vi "Read Instrument Configuration.vi"(8 "error in":errorcluster, 10 "Module Name":string, 11 "Instrument Config File Path":path) -> (0 "error out":errorcluster, 2 "Instrument Config":T1)   [LabVIEW 2023, in "Instrument Config.lvlib"]
uses:
  Instrument Config.lvlib
  <vilib>/Utility/config.llb/Read Key (String).vi
  <vilib>/Utility/config.llb/NI_LVConfig.lvlib
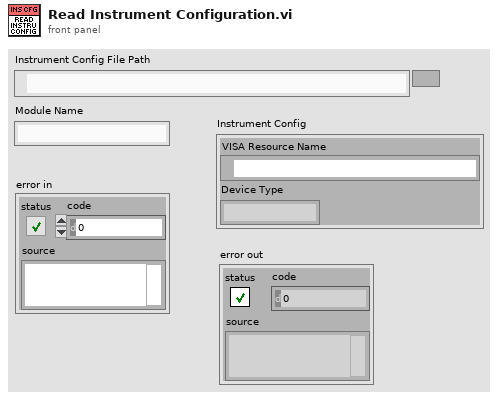
[diagram p1: front panel]
types:
  T1 = cluster{"VISA Resource Name":refnum<visa-resource-name>, "Device Type":string}
  T2 = typedef "NI_LVConfig.lvlib/Config Data RefNum.ctl" = refnum<k1>
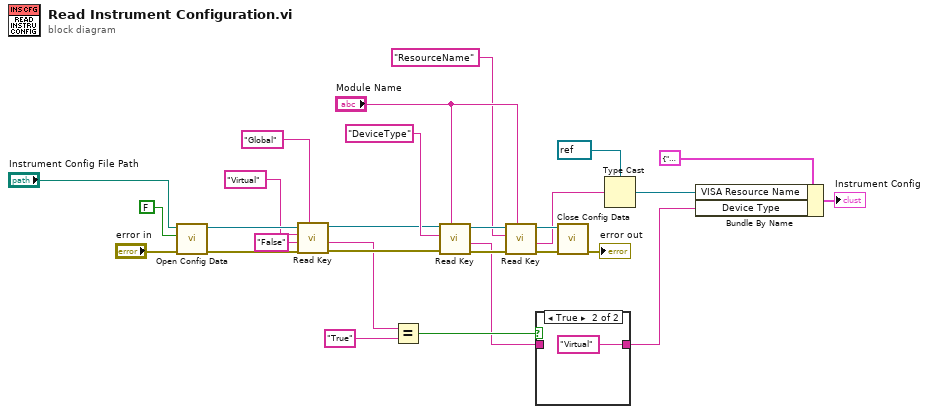
[diagram p0: block diagram]
diagram:
  n1 = call <vilib>:"Open Config Data.vi"("error in (no error)"="error in", "create file if necessary (T)"=FALSE, "configuration file path"="Instrument Config File Path") -> ("error out"=w10:errorcluster, "refnum"=w12:T2)  [unwired: 6 in, 1 out]
  n2 = call-poly <vilib>:"Read Key.vi"("section"="Global", "error in (no error)"=w10, "default value"="False", "key"="Virtual", "refnum"=w12) -> ("error out"=w9:errorcluster, "value"=w5:string, "refnum out"=w11:T2)  [unwired: 3 in, 1 out]
  n3 = Equal?(x=w5, y="True" ("regular expression")) -> (x = y?=w4:bool)
  n4 = call-poly <vilib>:"Read Key.vi"("section"="Module Name", "error in (no error)"=w9, "key"="DeviceType", "refnum"=w11) -> ("error out"=w28:errorcluster, "value"=w3:string, "refnum out"=w27:T2)  [unwired: 4 in, 1 out]
  n5 = call-poly <vilib>:"Read Key.vi"("section"="Module Name", "error in (no error)"=w28, "key"="ResourceName", "refnum"=w27) -> ("error out"=w26:errorcluster, "value"=w17:string, "refnum out"=w25:T2)  [unwired: 4 in, 1 out]
  n6 = case shown="True" w4 {
    tunnel: w3 -> [w29 _]
    tunnel: [w29 "Virtual"] -> w2
    frame False {
    }
    frame True {
    }
  }
  n7 = call <vilib>:"Close Config Data.vi"("error in (no error)"=w26, "refnum"=w25) -> ("error out"=→"error out":errorcluster)  [unwired: 8 in, 1 out]
  n8 = Type Cast(type=refnum<visa-resource-name> refnum ("VISA resource name"), x=w17) -> (*(type *) &x=w23:refnum<visa-resource-name>)
  n9 = Bundle By Name(cluster=T1 {"VISA Resource Name"="", "Device Type"=""} ("Instrument Config"), "VISA Resource Name"=w23, "Device Type"=w2) -> (→"Instrument Config":T1)
